vi "Obshee.vi"() -> ()   [LabVIEW 2016]
panel:
  in  "Cancel Button":bool
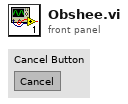
[diagram p1: front panel]
types:
  T1 = enum32{"Invalid", "Standard", "Closed", "Hidden", "Minimized", "Maximized"}
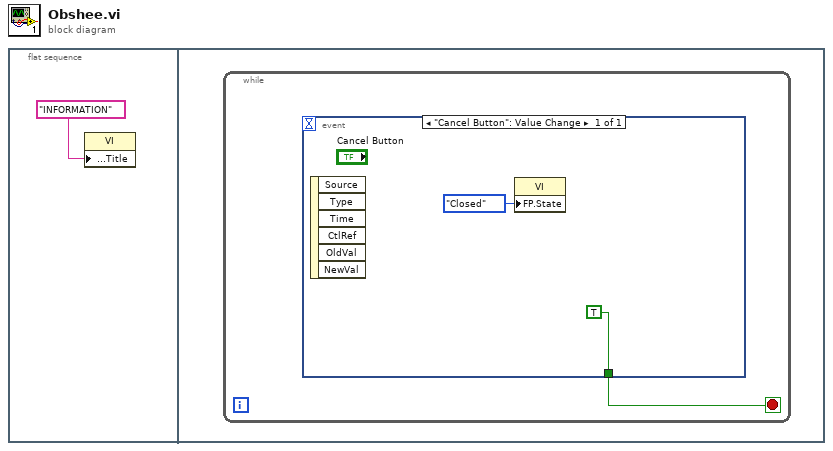
[diagram p0: block diagram]
diagram:
  n1 = flat-sequence {
    frame #0 {
      n2 = property class="VI"("Front Panel.Title"="INFORMATION" ("Front Panel Window:Title")) -> ()  [unwired: 2 in, 2 out]
    }
    frame #1 {
      n3 = while {
        stop <- w2 stop-if-true
        n4 = event shown="[0] \"Cancel Button\": Value Change" {
          selector: _ -> [_]
          dyn-events: _ -> [_]
          timeout: _ -> [_]
          tunnel: [TRUE] -> w2
          event "Cancel Button": Value Change {
            n5 = event-data() -> ()  [unwired: 1 in, 6 out]
            n6 = property class="VI"("FP.State"=T1."Closed" ("Front Panel Window:State")) -> ()  [unwired: 2 in, 2 out]
          }
        }
      }
    }
  }
